vi "Post Batch.vi"(8 "error in":errorcluster, 10 "Test Result In":T2, 11 "CalCfg File In":T1) -> (0 "error out":errorcluster, 1 "Pass":bool, 2 "Test Result Out":T2, 3 "CalCfg File Out":T1, 4 "String":string)   [LabVIEW 2020, in "GUCalibration2.lvlib"]
uses:
  GUCalibration2.lvlib
  Controls/Test Result.ctl
  Controls/Site Data Element.ctl
  Controls/Site Raw Data Element.ctl
  Controls/User Facing Msg Enum.ctl
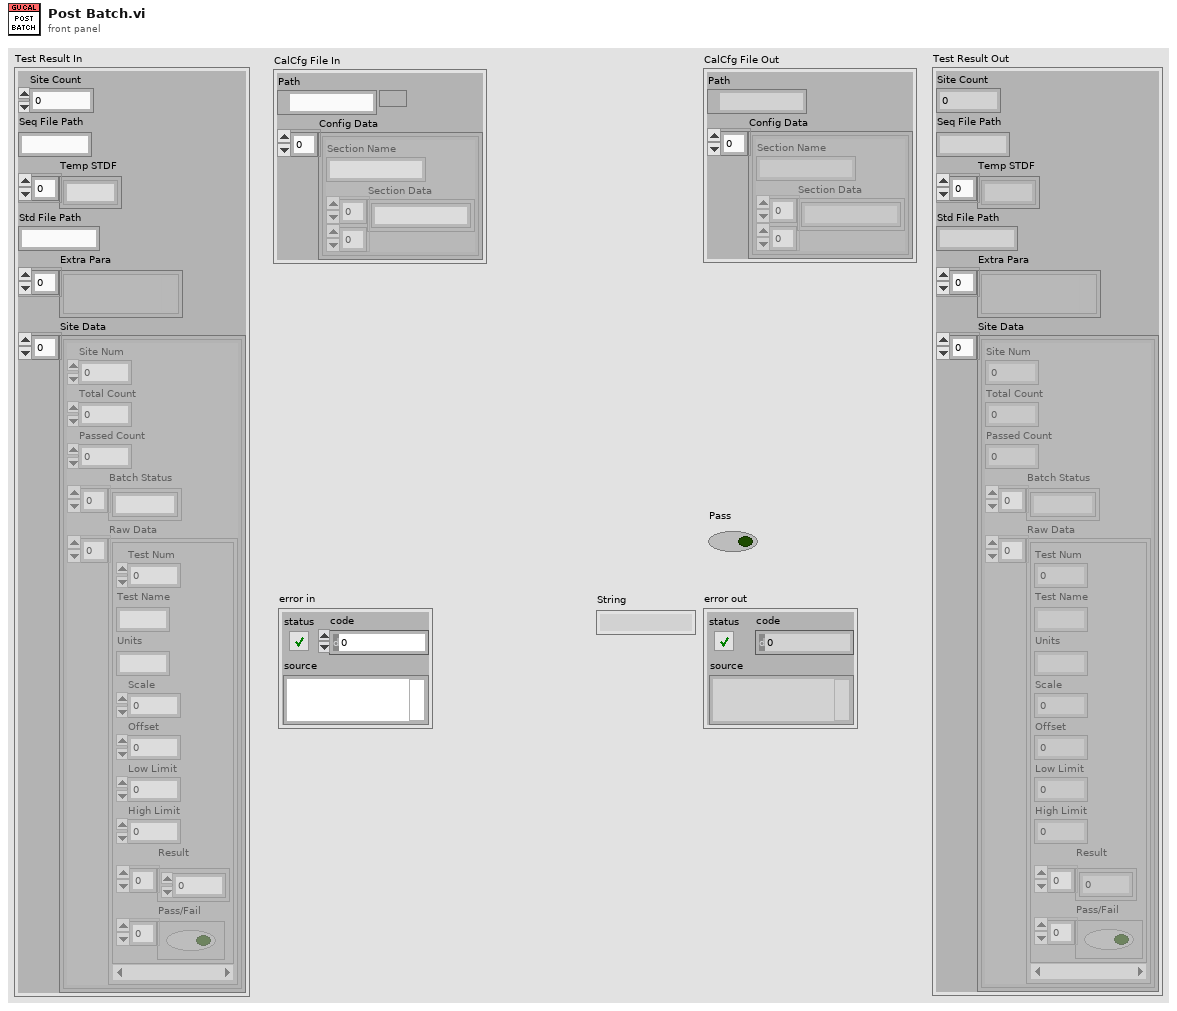
[diagram p1: front panel]
types:
  T1 = cluster{"Path":path, "Config Data":cluster{"Section Name":string, "Section Data":string[][]}[]}
  T2 = typedef "GUCalibration2.lvlib/Test Result.ctl" = cluster{"Site Count":i32, "Seq File Path":string, "Temp STDF":string[], "Std File Path":string, "Extra Para":variant[], "Site Data":T3[]}
  T3 = typedef "GUCalibration2.lvlib/Site Data Element.ctl" = cluster{"Site Num":i32, "Total Count":i32, "Passed Count":i32, "Batch Status":string[], "Raw Data":T4[]}
  T4 = typedef "GUCalibration2.lvlib/Site Raw Data Element.ctl" = cluster{"Test Num":u32, "Test Name":string, "Units":string, "Scale":i8, "Offset":dbl, "Low Limit":dbl, "High Limit":dbl, "Result":dbl[], "Pass/Fail":bool[]}
  T5 = typedef "GUCalibration2.lvlib/User Facing Msg Enum.ctl" = enum16{"Invalid GU Number", "Select More GU", "Exceptional Lot End", "Not All Sites Test", "GU Arrange Error", "Put GU In Sites", "No Cal Site Offset Msg"}
  T6 = cluster{"Section Name":string, "Section Data":string[][]}[]
  T7 = typedef "GUCalibration2.lvlib/Config Data Type.ctl" = cluster{"Cal Type":i32, "Curr Batch Index":i32, "Loop Count Per GU":i32, "Min Num of Pass GUs Per Site":i32, "Is Calibration":bool, "Batch Iteration Done":bool, "Cal Abort":bool, "Update Offset":bool, "Cal Check Pass":bool, "Cal End":bool, "Enabled Site":i32[], "GU Selected":i32[], "All Available GU":i32[], "GU Arrange":i32[][], "Batch Test Count":i32[][], "Batch Test Result":string[][], "Curr Batch":i32[], "Curr Batch Test Count":i32[], "Curr Batch Target Count":i32[], "Curr Batch Test Result":string[]}
  T8 = cluster{"Check Limit":bool[], "Cal Limit":bool[], "Cal GU Pass":bool[][], "Check GU Pass":bool[][], "Site Num":i32[], "GU Num":string[][]}
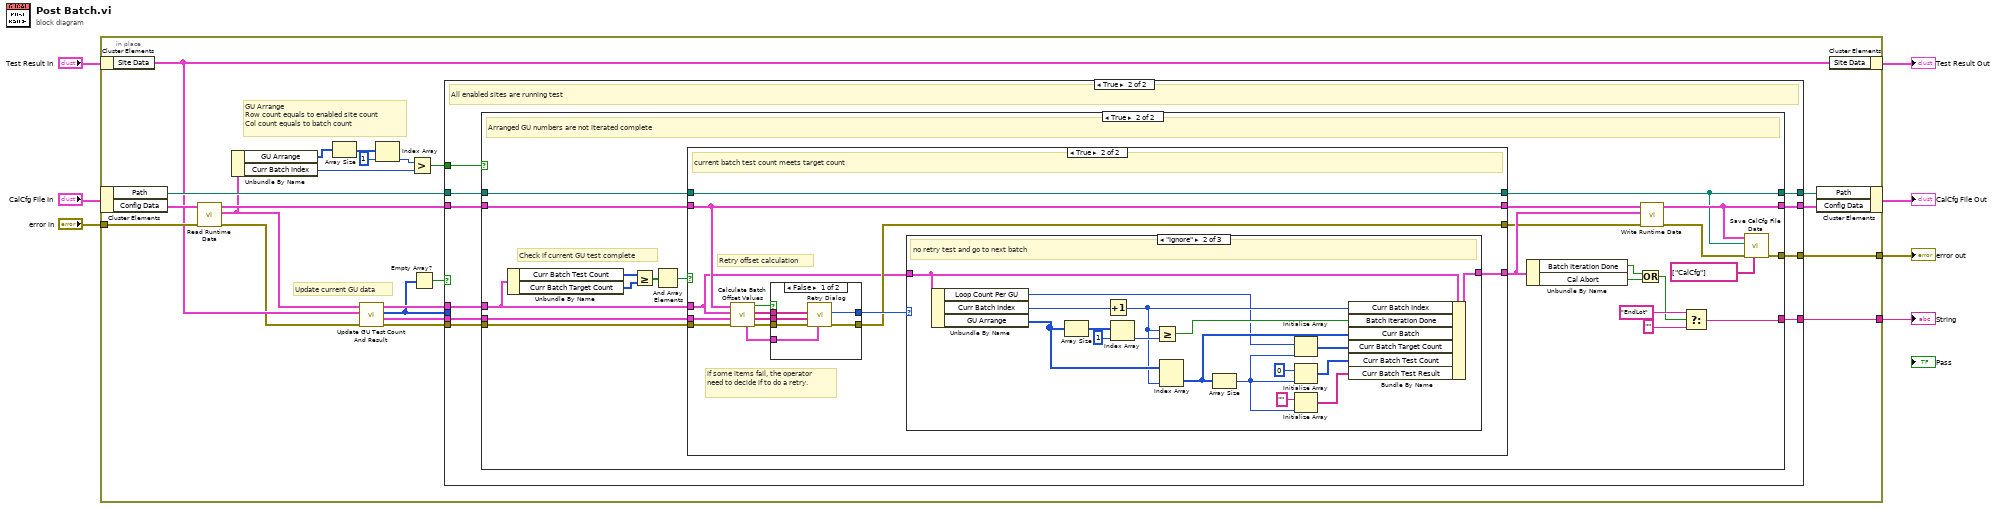
[diagram p0: block diagram]
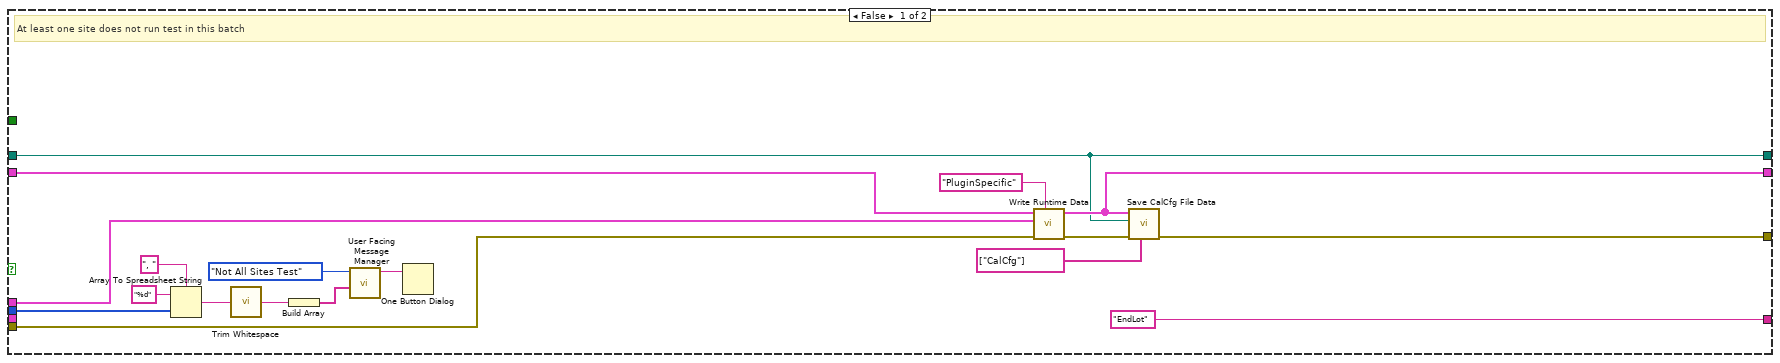
[diagram p2: hidden frame]
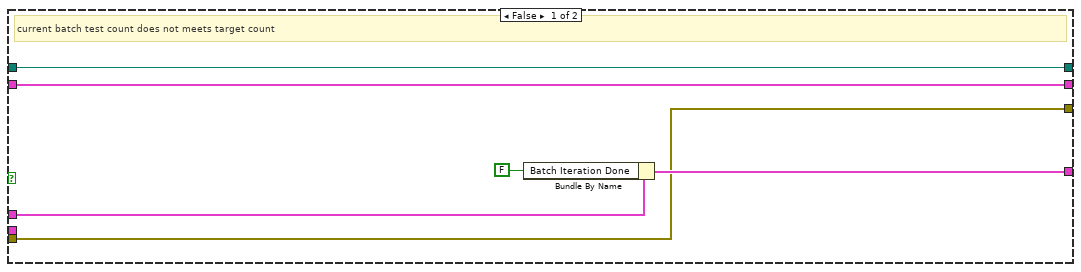
[diagram p4: hidden frame]
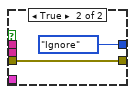
[diagram p5: hidden frame]
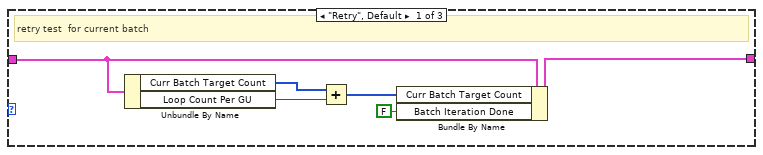
[diagram p6: hidden frame]
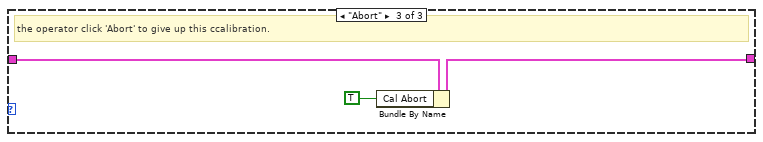
[diagram p7: hidden frame]
diagram:
  n1 = in-place {
    in-place-border: "error in" -> [w28]
    in-place-border: [w25] -> w6
    in-place-border: [w16] -> w3
    # "GU Arrange \nRow count equals to enabled site count\nCol count equals to batch count"
    # "Update current GU data"
    n2 = in-place-cluster #1("Test Result In") -> ("Site Data"=w13:T3[])
    n3 = in-place-cluster #2("CalCfg File In") -> ("Path"=w24:path, "Config Data"=w29:T6)
    n4 = call "Read Runtime Data.vi"("error in"=w28, "Config File Data In"=w29) -> ("error out"=w12:errorcluster, "Runtime Data Out"=w15:T7, "Config Data Out"=w27:T6)  [unwired: 7 in]
    n5 = Unbundle By Name(w15) -> ("GU Arrange"=w21:i32[][], "Curr Batch Index"=w19:i32)
    n6 = Array Size(array=w21) -> (size(s)=w23:i32[])
    n7 = call "Update GU Test Count And Result.vi"("error in"=w12, "Site Data In"=w13, "Runtime Data In"=w15) -> ("error out"=w11:errorcluster, "Site Data Out"=w8:T3[], "Sites Without Testing"=w9:i32[], "Runtime Data Out"=w14:T7)  [unwired: 5 in]
    n8 = Index Array(array=w23, index=1) -> (element=w20:i32)
    n9 = Greater?(x=w20, y=w19) -> (0:w17:bool)
    n10 = Empty Array?(array=w9) -> (empty?=w10:bool)
    n11 = case shown="True" w10 {
      tunnel: w27 -> [w38 w57]
      tunnel: [w35 w56] -> w26
      tunnel: [w32 w55] -> w25
      tunnel: w24 -> [w34 w54]
      tunnel: [w34 w53] -> w18
      tunnel: w17 -> [_ w52]
      tunnel: ["EndLot" ("f") w51] -> w16
      tunnel: w14 -> [w36 w50]
      tunnel: w11 -> [w39 w49]
      tunnel: w9 -> [w47 _]
      tunnel: w8 -> [_ w48]
      frame False {
        # "At least one site does not run test in this batch"
        n12 = Array To Spreadsheet String(delimiter (Tab)=", ", array=w47, 3:"%d" ("format string")) -> (spreadsheet string=w45:string)
        n13 = call <vilib>:"Trim Whitespace.vi"("string"=w45) -> ("trimmed string"=w44:string)  [unwired: 1 in]
        n14 = Build Array(w44) -> (w43:string[])
        n15 = call "User Facing Message Manager.vi"("Variable Msg"=w43, "User Facing Msg"=User_Facing_Msg_Enum."Not All Sites Test") -> ("User Facing Msg Out"=w30:string)  [unwired: 7 in, 2 out]
        n16 = One Button Dialog(message=w30) -> ()  [unwired: 1 in, 1 out]
        n17 = call "Write Runtime Data.vi"("Section Name"="PluginSpecific", "error in"=w39, "Runtime Data In"=w36, "Config File Data In"=w38) -> ("error out"=w33:errorcluster, "Config Data Out"=w35:T6)  [unwired: 5 in, 1 out]
        n18 = call "Save CalCfg File Data.vi"("Matric Section"=string[] ["CalCfg"], "error in"=w33, "File Path"=w34, "Config Data"=w35) -> ("error out"=w32:errorcluster)  [unwired: 7 in]
      }
      frame True {
        # "All enabled sites are running test"
        n19 = case shown="True" w52 {
          tunnel: w49 -> [w58 w66]
          tunnel: w57 -> [w59 w67]
          tunnel: [w59 w78] -> w56
          tunnel: [w58 w76] -> w55
          tunnel: w54 -> [w60 w69]
          tunnel: w50 -> [_ w64]
          tunnel: [w60 w70] -> w53
          tunnel: [_ w73] -> w51
          tunnel: w48 -> [_ w65]
          frame False {
            # "Ignore testing data here"
            # "Arranged GU numbers are iterated complete"
          }
          frame True {
            # "Check if current GU test complete"
            # "Arranged GU numbers are not iterated complete"
            n20 = Unbundle By Name(w64) -> ("Curr Batch Test Count"=w83:i32[], "Curr Batch Target Count"=w82:i32[])
            n21 = Greater Or Equal?(x=w83, y=w82) -> (x >= y?=w81:bool[])
            n22 = And Array Elements(Boolean array=w81) -> (logical AND=w80:bool)
            n23 = case shown="True" w80 {
              tunnel: [w89 w102] -> w72
              tunnel: [w87 w97] -> w71
              tunnel: w67 -> [w87 w97]
              tunnel: [w86 w101] -> w70
              tunnel: w69 -> [w86 w101]
              tunnel: [w84 w99] -> w68
              tunnel: w66 -> [w84 w95]
              tunnel: w65 -> [_ w98]
              tunnel: w64 -> [w85 w96]
              frame False {
                # "current batch test count does not meets target count"
                n24 = Bundle By Name(cluster=w85, "Batch Iteration Done"=FALSE ("Calibration End")) -> (w89:T7)
              }
              frame True {
                # "Retry offset calculation"
                # "if some items fail, the operator need to decide if to do a retry."
                # "current batch test count meets target count"
                n25 = call "Calculate Batch Offset Values.vi"("error in"=w95, "Site Data"=w98, "Cal Runtime Cfg"=w96, "Config Data"=w97) -> ("error out"=w94:errorcluster, "Data String"=w91:string[][], "Col Header String"=w92:string[], "All Items Pass?"=w93:bool, "Limit Status"=w90:T8)  [unwired: 3 in]
                n26 = case shown="False" w93 {
                  tunnel: w94 -> [w108 w110]
                  tunnel: w92 -> [w107 _]
                  tunnel: [w106 w110] -> w99
                  tunnel: [w105 enum16{"Retry", "Ignore", "Abort"}."Ignore" ("Next Action")] -> w100
                  tunnel: w91 -> [w104 _]
                  tunnel: w90 -> [w103 _]
                  frame False {
                    n27 = call "Retry Dialog.vi"("Limit Status"=w103, "error in"=w108, "Data String"=w104, "Col Header String"=w107) -> ("error out"=w106:errorcluster, "Next Action"=w105:enum16{"Retry", "Ignore", "Abort"})  [unwired: 6 in]
                  }
                  frame True {
                  }
                }
                n28 = case shown="\"Ignore\"" w100 {
                  tunnel: w96 -> [w116 w131 w136]
                  tunnel: [w115 w127 w135] -> w102
                  frame "Retry", Default {
                    # "retry test  for current batch"
                    n29 = Unbundle By Name(w116) -> ("Curr Batch Target Count"=w114:i32[], "Loop Count Per GU"=w113:i32)
                    n30 = Add(x=w114, y=w113) -> (x+y=w112:i32[])
                    n31 = Bundle By Name(cluster=w116, "Curr Batch Target Count"=w112, "Batch Iteration Done"=FALSE ("Calibration End")) -> (w115:T7)
                  }
                  frame "Ignore" {
                    # "no retry test and go to next batch"
                    n32 = Unbundle By Name(w131) -> ("Loop Count Per GU"=w122:i32, "Curr Batch Index"=w130:i32, "GU Arrange"=w126:i32[][])
                    n33 = Array Size(array=w126) -> (size(s)=w133:i32[])
                    n34 = Increment(x=w130) -> (x+1=w125:i32)
                    n35 = Index Array(array=w133, index=1) -> (element=w129:i32)
                    n36 = Greater Or Equal?(x=w125, y=w129) -> (x >= y?=w128:bool)
                    n37 = Index Array(array=w126, index (col)=w125) -> (element=w124:i32[])  [unwired: 1 in]
                    n38 = Array Size(array=w124) -> (size(s)=w119:i32)
                    n39 = Initialize Array(w122, w119) -> (w123:i32[])
                    n40 = Initialize Array(0 ("element"), w119) -> (w120:i32[])
                    n41 = Initialize Array("" ("F button name (\"Cancel\")"), w119) -> (w118:string[])
                    n42 = Bundle By Name(cluster=w131, "Curr Batch Index"=w125, "Batch Iteration Done"=w128, "Curr Batch"=w124, "Curr Batch Target Count"=w123, "Curr Batch Test Count"=w120, "Curr Batch Test Result"=w118) -> (w127:T7)
                  }
                  frame "Abort" {
                    # "the operator click 'Abort' to give up this ccalibration."
                    n43 = Bundle By Name(cluster=w136, "Cal Abort"=TRUE) -> (w135:T7)
                  }
                }
              }
            }
            n44 = Unbundle By Name(w72) -> ("Batch Iteration Done"=w63:bool, "Cal Abort"=w62:bool)
            n45 = Or(x=w63, y=w62) -> (x .or. y?=w61:bool)
            n46 = call "Write Runtime Data.vi"("error in"=w68, "Runtime Data In"=w72, "Config File Data In"=w71) -> ("error out"=w77:errorcluster, "Config Data Out"=w78:T6)  [unwired: 6 in, 1 out]
            n47 = Select(t="EndLot" ("String"), s=w61, f="") -> (s? t:f=w73:string)
            n48 = call "Save CalCfg File Data.vi"("Matric Section"=string[] ["CalCfg"], "error in"=w77, "File Path"=w70, "Config Data"=w78) -> ("error out"=w76:errorcluster)  [unwired: 7 in]
          }
        }
      }
    }
    n49 = in-place-cluster #2("Path"=w18, "Config Data"=w26) -> (→"CalCfg File Out":T1)
    n50 = in-place-cluster #1("Site Data"=w13) -> (→"Test Result Out":T2)
  }
  "error out" <- w6
  "String" <- w3
